vi "XMLExtractRowData.vi"(11 "Rows":string[](array[string])) -> (2 "Contents":string[][](array[string]), 3 "Cell Type Data":string[][](array[string]))   [LabVIEW 2014]
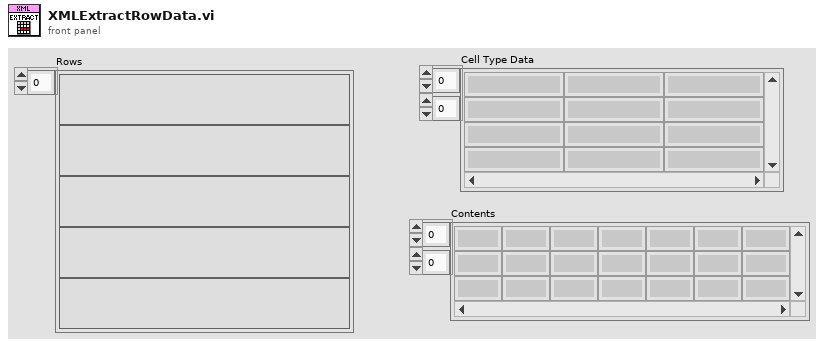
[diagram p1: front panel]
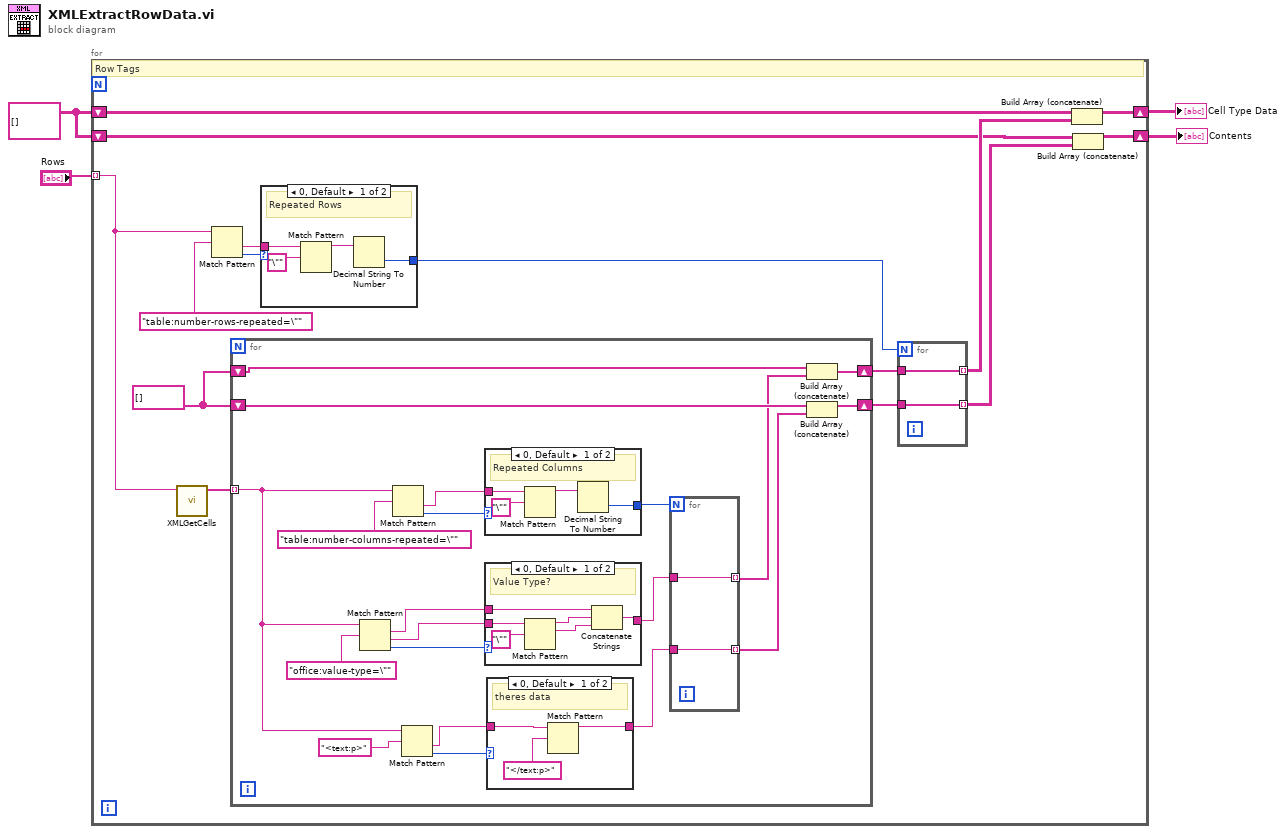
[diagram p0: block diagram]
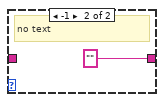
[diagram p2: hidden frame]
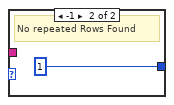
[diagram p3: hidden frame]
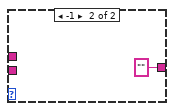
[diagram p4: hidden frame]
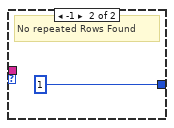
[diagram p5: hidden frame]
diagram:
  w3 = string[][] []
  n1 = for {
    tunnel: "Rows" -> [w17] mode=indexing
    shift-right: [w8] -> w1
    shift-left: w3 -> [w13]
    shift-right: [w5] -> w2
    shift-left: w3 -> [w7]
    w14 = string[] []
    # "Row Tags"
    n2 = call "XMLGetCells.vi"("XML"=w17) -> ("Cells"=w16:string[])  [unwired: 10 in]
    n3 = Match Pattern(string=w17, regular expression="table:number-rows-repeated=\"") -> (after substring=w18:string, offset past match=w19:i32)  [unwired: 1 in, 2 out]
    n4 = for {
      tunnel: w16 -> [w32] mode=indexing
      shift-right: [w23] -> w12
      shift-left: w14 -> [w27]
      shift-right: [w22] -> w10
      shift-left: w14 -> [w26]
      n5 = Match Pattern(string=w32, regular expression="office:value-type=\"") -> (match substring=w36:string, after substring=w37:string, offset past match=w40:i32)  [unwired: 1 in, 1 out]
      n6 = Match Pattern(string=w32, regular expression="table:number-columns-repeated=\"") -> (after substring=w31:string, offset past match=w38:i32)  [unwired: 1 in, 2 out]
      n7 = Match Pattern(string=w32, regular expression="<text:p>") -> (after substring=w30:string, offset past match=w29:i32)  [unwired: 1 in, 2 out]
      n8 = case shown="0, Default" w38 {
        tunnel: w31 -> [w51 _]
        tunnel: [w48 1] -> w35
        frame 0, Default {
          # "Repeated Columns"
          n9 = Match Pattern(string=w51, regular expression="\"") -> (before substring=w49:string)  [unwired: 1 in, 3 out]
          n10 = Decimal String To Number(string=w49) -> (number=w48:i32)  [unwired: 2 in, 1 out]
        }
        frame -1 {
          # "No repeated Rows Found"
        }
      }
      n11 = case shown="0, Default" w40 {
        tunnel: w37 -> [w58 _]
        tunnel: w36 -> [w56 _]
        tunnel: [w53 ""] -> w34
        frame 0, Default {
          # "Value Type?"
          n12 = Match Pattern(string=w58, regular expression="\"") -> (before substring=w55:string, match substring=w54:string)  [unwired: 1 in, 2 out]
          n13 = Concatenate Strings(w56, w55, w54) -> (w53:string)
        }
        frame -1 {
        }
      }
      n14 = case shown="0, Default" w29 {
        tunnel: w30 -> [w44 _]
        tunnel: [w42 ""] -> w28
        frame 0, Default {
          # "theres data"
          n15 = Match Pattern(string=w44, regular expression="</text:p>") -> (before substring=w42:string)  [unwired: 1 in, 3 out]
        }
        frame -1 {
          # "no text"
        }
      }
      n16 = for {
        N: w35 -> [_]
        tunnel: w34 -> [w47]
        tunnel: w28 -> [w46]
        tunnel: [w47] -> w25 mode=indexing
        tunnel: [w46] -> w24 mode=indexing
      }
      n17 = Build Array (concatenate)(w27, w25) -> (w23:string[])
      n18 = Build Array (concatenate)(w26, w24) -> (w22:string[])
    }
    n19 = case shown="0, Default" w19 {
      tunnel: w18 -> [w63 _]
      tunnel: [w60 1] -> w11
      frame 0, Default {
        # "Repeated Rows"
        n20 = Match Pattern(string=w63, regular expression="\"") -> (before substring=w61:string)  [unwired: 1 in, 3 out]
        n21 = Decimal String To Number(string=w61) -> (number=w60:i32)  [unwired: 2 in, 1 out]
      }
      frame -1 {
        # "No repeated Rows Found"
      }
    }
    n22 = for {
      N: w11 -> [_]
      tunnel: w12 -> [w21]
      tunnel: w10 -> [w20]
      tunnel: [w21] -> w9 mode=indexing
      tunnel: [w20] -> w6 mode=indexing
    }
    n23 = Build Array (concatenate)(w13, w9) -> (w8:string[][])
    n24 = Build Array (concatenate)(w7, w6) -> (w5:string[][])
  }
  "Cell Type Data" <- w1
  "Contents" <- w2
